vi "fgv_StimTrigLive-Setup.vi"(0 "Function":enum16{"Intialize", "Write", "Read", "Clear"}(ring), 5 "Live stim.trig.enable":bool, 7 "Live stim.trig.period (sec)":dbl, 9 "Live stim.trig.width (ms)":dbl, 11 "error in (no error)":errorcluster) -> (6 "Live stim.trig.enable":bool, 8 "Live stim.trig.period (sec)":dbl format="%#_7f", 10 "Live stim.trig.width (ms)":dbl, 15 "error out":errorcluster)   [LabVIEW 2020]
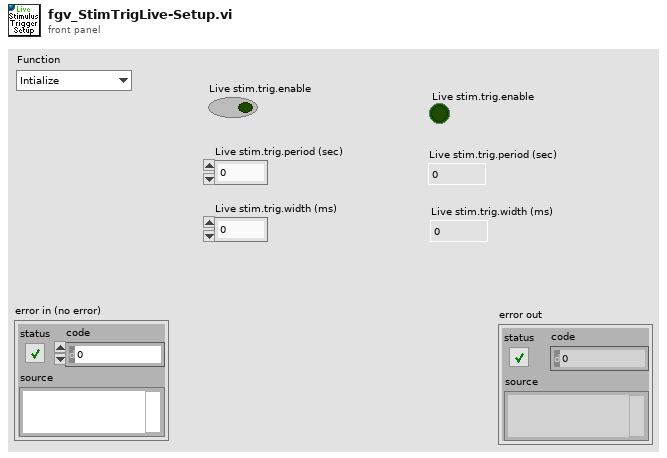
[diagram p1: front panel]
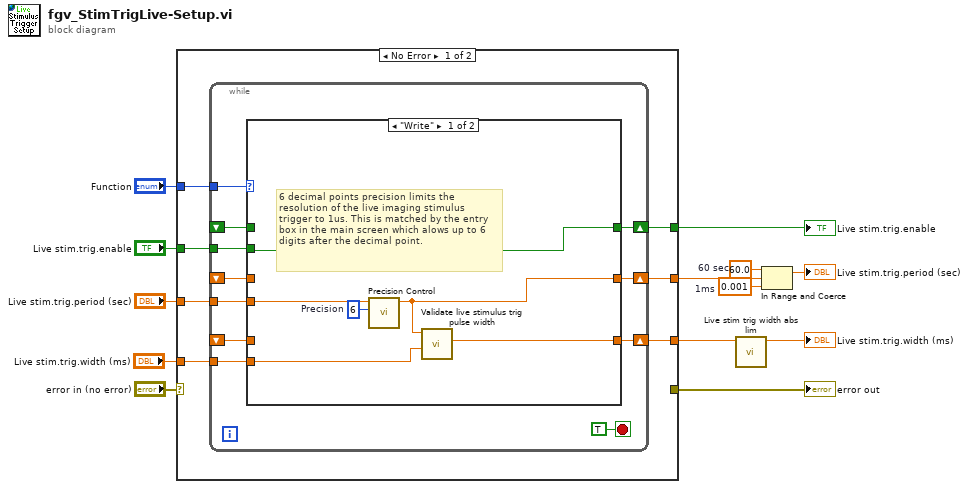
[diagram p0: block diagram]
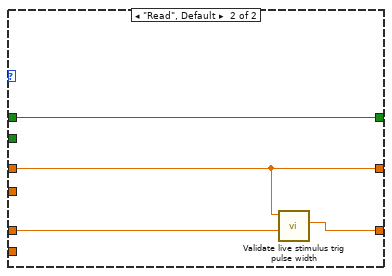
[diagram p2: hidden frame]
diagram:
  w6 = 60.0  # 60 sec
  w5 = 0.001  # 1ms
  n1 = case shown="No Error" "error in (no error)" {
    selector: "error in (no error)" -> [_ w45]
    tunnel: [_ w45] -> w12
    tunnel: "Function" -> [w20 _]
    tunnel: "Live stim.trig.enable" -> [w19 w44]
    tunnel: [w18 w44] -> w9
    tunnel: "Live stim.trig.period (sec)" -> [w17 w43]
    tunnel: [w16 w43] -> w3
    tunnel: "Live stim.trig.width (ms)" -> [w15 w42]
    tunnel: [w14 w42] -> w1
    frame No Error {
      n2 = while {
        tunnel: w20 -> [w30]
        tunnel: w19 -> [w29]
        shift-right: [w28] -> w18
        shift-left: _ -> [w27]
        tunnel: w17 -> [w25]
        shift-right: [w26] -> w16
        shift-left: _ -> [w24]
        tunnel: w15 -> [w22]
        shift-right: [w23] -> w14
        shift-left: _ -> [w21]
        stop <- TRUE stop-if-true
        n3 = case shown="\"Write\"" w30 {
          tunnel: [w37 w41] -> w28
          tunnel: w29 -> [w37 _]
          tunnel: w27 -> [_ w41]
          tunnel: [w33 w40] -> w26
          tunnel: w25 -> [w34 _]
          tunnel: w24 -> [_ w40]
          tunnel: [w35 w38] -> w23
          tunnel: w22 -> [w36 _]
          tunnel: w21 -> [_ w39]
          frame "Write" {
            w32 = u8 6  # Precision
            # "6 decimal points precision limits the resolution of the live imaging stimulus trigger to 1us. This is matched by the entry box in the main screen which alows up to 6 digits after the decimal point."
            n4 = call <userlib>:"Precision Control.vi"("Precision"=w32, "Input Value"=w34) -> ("Output Value"=w33:dbl)  [unwired: 8 in, 1 out]
            n5 = call "Validate live stimulus trig pulse width.vi"("Requested trigger pulse width (ms)"=w36, "Trigger period (sec)"=w33) -> ("Live imaging. stimulus trigger pulse width (ms)"=w35:dbl)  [unwired: 9 in]
          }
          frame "Read", Default {
            n6 = call "Validate live stimulus trig pulse width.vi"("Requested trigger pulse width (ms)"=w39, "Trigger period (sec)"=w40) -> ("Live imaging. stimulus trigger pulse width (ms)"=w38:dbl)  [unwired: 9 in]
          }
        }
      }
    }
    frame Error {
    }
  }
  "error out" <- w12
  "Live stim.trig.enable" <- w9
  n7 = call "Live stim trig width abs lim.vi"("Live stim.trig.width (ms)"=w1) -> ("Live stim.trig.width (ms)"=→"Live stim.trig.width (ms)":dbl)  [unwired: 10 in]
  n8 = In Range and Coerce(upper limit=w6, x=w3, lower limit=w5) -> (coerced(x)=→"Live stim.trig.period (sec)":dbl)  [unwired: 1 out]
